vi "ColorDetect_V1.vi"(8 "error in (no error)":errorcluster, 9 "Color Upper":T1, 10 "Color Lower":T1, 11 "new picture":picture) -> (0 "error out":errorcluster, 1 "found (X,Y,R)":u32[][](array[numeric]), 2 "image":u8[][](array[numeric]), 3 "out picture":picture)   [LabVIEW 2014, in "QwaveSys RPi Training Library.lvlib"]
uses:
  <vilib>/Q-Wave Systems/QwaveSys RPi Package 2.0/Addons/QwaveSys RPi Training Library.lvlib
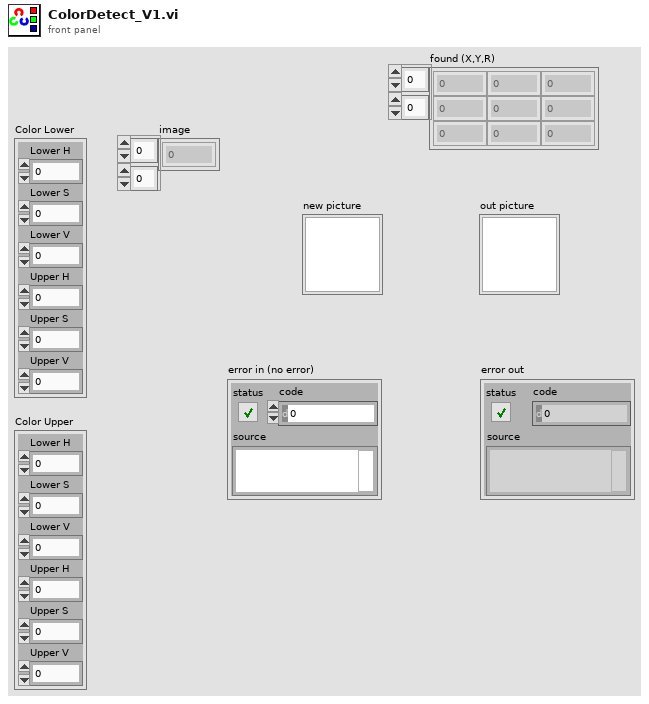
[diagram p1: front panel]
types:
  T1 = cluster{"Lower H":u8, "Lower S":u8, "Lower V":u8, "Upper H":u8, "Upper S":u8, "Upper V":u8}
  T2 = cluster{"Width":u16, "Style":enum32{"Solid", "Dash", "Dot", "DashDot", "DashDotDot"}}
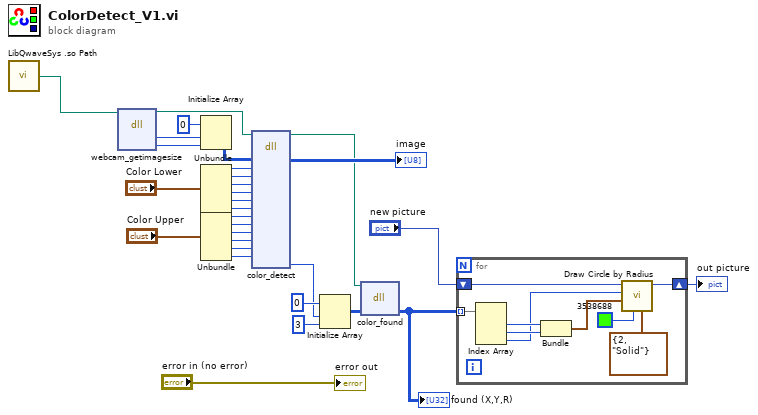
[diagram p0: block diagram]
diagram:
  n1 = call <vilib>:"LibQwaveSys .so Path.vi"() -> ("Lib QwaveSys .so Path"=w3:path)  [unwired: 5 in]
  n2 = dll-call lib="libqwavesys.so" fn="webcam_getimagesize"(path in=w3) -> (path out=w2:path, "rows"=w29:i32, "cols"=w30:i32)  [unwired: 5 in, 1 out]
  n3 = Initialize Array(u8 0 ("element"), w29, w30) -> (w28:u8[][])
  n4 = Unbundle("Color Lower") -> ("Lower H"=w15:u8, "Lower S"=w16:u8, "Lower V"=w17:u8, "Upper H"=w18:u8, "Upper S"=w19:u8, "Upper V"=w20:u8)
  n5 = Unbundle("Color Upper") -> ("Lower H"=w22:u8, "Lower S"=w23:u8, "Lower V"=w24:u8, "Upper H"=w25:u8, "Upper S"=w26:u8, "Upper V"=w27:u8)
  n6 = dll-call lib="libqwavesys.so" fn="color_detect"(path in=w2, "image"=w28, "Alower_h"=w15, "Alower_s"=w16, "Alower_v"=w17, "Aupper_h"=w18, "Aupper_s"=w19, "Aupper_v"=w20, "Blower_h"=w22, "Blower_s"=w23, "Blower_v"=w24, "Bupper_h"=w25, "Bupper_s"=w26, "Bupper_v"=w27) -> (path out=w1:path, "image"=→"image":u8[][], "found"=w8:i32)  [unwired: 16 in, 1 out]
  n7 = Initialize Array(u32 0 ("element"), w8, 3 ("dimension size")) -> (w9:u32[][])
  n8 = dll-call lib="libqwavesys.so" fn="color_found"(path in=w1, "found"=w9) -> ("found"=w6:u32[][])  [unwired: 3 in, 2 out]
  "found (X,Y,R)" <- w6
  n9 = for {
    tunnel: w6 -> [w37] mode=indexing
    shift-right: [w31] -> w4
    shift-left: "new picture" -> [w32]
    n10 = Index Array(array=w37) -> (element #1=w36:u32, element #2=w35:u32, element #3=w34:u32)  [unwired: 3 in]
    n11 = Bundle(w36, w35) -> (w39:cluster{u32, u32})  [unwired: 1 in]
    n12 = call <vilib>:"Draw Circle by Radius.vi"("pen"=T2 {"Width"=2, "Style"=enum."Solid"}, "color(black)"=u32 3538688, "pixel center"=w39, "radius"=w34, "picture"=w32) -> ("new picture"=w31:picture)  [unwired: 6 in]
  }
  "out picture" <- w4
  "error out" <- "error in (no error)"
